vi "U6 Single EI-1050 Example.vi"() -> ()   [LabVIEW 2021]
panel:
  in  "stop":bool
  out "ms per iteration":u32
  out "RH A [%]":dbl format="%.6f"
  out "Temp A [degC]":dbl format="%.6f"
  out "Error Message":string
  out "error out":errorcluster
  # "Reads temperature and humidity from an EI-1050 probe:\n\nEI-1050 Connections:\nRed (Power)         FIO3\nBlack (Ground)     GND\nGreen (Data)        FIO0\nWhite (Clock)       FIO1\nBrown (Enable)    FIO3"
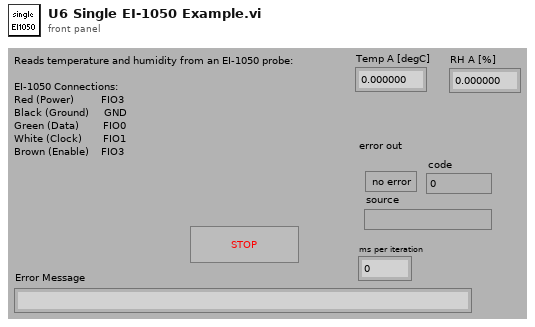
[diagram p1: front panel]
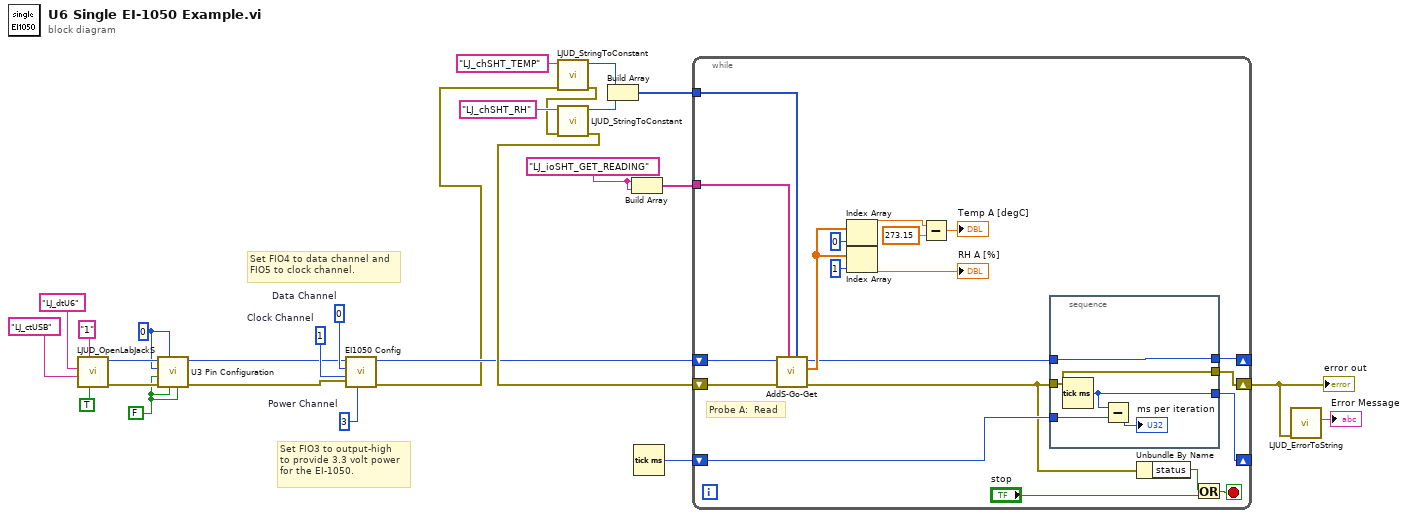
[diagram p0: block diagram]
diagram:
  w5 = 0  # Data Channel
  w6 = 1  # Clock Channel
  w7 = 3  # Power Channel
  w8 = FALSE ("Enable DAC1")
  w9 = 0 ("FIO/EIO Analog Enable")
  w22 = "LJ_ioSHT_GET_READING" ("IOType")
  # "Set FIO4 to data channel and\nFIO5 to clock channel."
  # "Set FIO3 to output-high\nto provide 3.3 volt power\nfor the EI-1050."
  n1 = call "LJUD_OpenLabJackS.vi"("FirstFound"=TRUE, "Address"="1", "ConnectionType"="LJ_ctUSB", "DeviceType"="LJ_dtU6") -> ("error out"=w10:errorcluster, "Handle"=w11:i32)  [unwired: 5 in, 1 out]
  n2 = call "U3 Pin Configuration.vi"("Enable Counter1"=w8, "Enable Counter0"=w8, "FIO/EIO Analog Enable"=w9, "error in"=w10, "Enable DAC1"=w8, "Number of Timers Enabled"=w9, "Handle In"=w11) -> ("error out"=w3:errorcluster, "Handle Out"=w4:i32)  [unwired: 3 in]
  n3 = call "EI1050 Config.vi"("Power Channel"=w7, "error in"=w3, "Clock Channel"=w6, "Data Channel"=w5, "Handle In"=w4) -> ("error out"=w1:errorcluster, "Handle Out"=w2:i32)  [unwired: 5 in]
  n4 = call "LJUD_StringToConstant.vi"("error in"=w1, "String"="LJ_chSHT_TEMP") -> ("error out"=w13:errorcluster, "Constant Number"=w21:i32)  [unwired: 8 in]
  n5 = call "LJUD_StringToConstant.vi"("error in"=w13, "String"="LJ_chSHT_RH") -> ("error out"=w12:errorcluster, "Constant Number"=w20:i32)  [unwired: 8 in]
  n6 = Build Array(w21, w20) -> (w16:i32[])
  n7 = Build Array(w22, w22) -> (w17:string[])
  n8 = Tick Count (ms)() -> (millisecond timer value=w15:u32)
  n9 = while {
    shift-left: w15 -> [w37]
    shift-right: [w40] -> _
    shift-left: w2 -> [w29]
    shift-right: [w38] -> _
    shift-left: w12 -> [w28]
    shift-right: [w39] -> w14
    tunnel: w16 -> [w33]
    tunnel: w17 -> [w32]
    stop <- w36 stop-if-true
    # "Probe A:  Read"
    n10 = call "AddS-Go-Get.vi"("Channels"=w33, "IOTypes"=w32, "error in"=w28, "Handle In"=w29) -> ("error out"=w30:errorcluster, "Values Read"=w45:dbl[], "Handle Out"=w31:i32)  [unwired: 5 in]
    n11 = Index Array(array=w45, index=0 ("Index")) -> (element=w42:dbl)
    n12 = Index Array(array=w45, index=1 ("Index")) -> (element=→"RH A [%]":dbl)
    n13 = Subtract(x=w42, y=273.15) -> (x-y=→"Temp A [degC]":dbl)
    n14 = stacked-sequence {
      tunnel: [w52] -> w40
      tunnel: w30 -> [w51]
      tunnel: [w51] -> w39
      tunnel: [w50] -> w38
      tunnel: w31 -> [w50]
      tunnel: w37 -> [w49]
      frame #0 {
        n15 = Tick Count (ms)() -> (millisecond timer value=w52:u32)
        n16 = Subtract(x=w52, y=w49) -> (x-y=→"ms per iteration":u32)
      }
    }
    n17 = Unbundle By Name(w30) -> ("status"=w35:bool)
    n18 = Or(x=w35, y="stop") -> (x .or. y?=w36:bool)
  }
  "error out" <- w14
  n19 = call "LJUD_ErrorToString.vi"("error in"=w14) -> ("String"=→"Error Message":string)  [unwired: 10 in]
